vi "KeyInCounterPosition.vi"() -> (1 "Counter Position output":dbl=950.0 min=0.0 max=2600.0 format="%.3f", 2 "Stepper Position":i32)   [LabVIEW 2020]
uses:
  Calibration/GlobalCalLampInfo.vi
  Globals and TypeDefs/gSpectrometer.vi
panel:
  in  "Reset":bool
  in  "Current Wavelength":dbl=703.2413 caption="Input Calibration Wavelength (nm)" format="%.4f"
  in  "Select WL":u16(ring)=5 caption="Select a Target Calibration Line" items=["808.2458  nm  ( Ne )", "794.3181  nm  ( Ne )", "743.8898  nm  ( Ne )", "724.5167  nm  ( Ne )", "717.3938  nm  ( Ne )", "703.2413  nm  ( Ne )", "692.9467  nm  ( Ne )", "671.7043  nm  ( Ne )", "667.8276  nm  ( Ne )", "659.8953  nm  ( Ne )", "653.2882  nm  ( Ne )", "650.6528  nm  ( Ne )", "640.2246  nm  ( Ne )", "638.2991  nm  ( Ne )", "633.4428  nm  ( Ne )", "632.8165  nm  ( Ne )", "579.2200  nm  ( Hg )", "577.1100  nm  ( Hg )", "546.2200  nm  ( Hg )", "435.9500  nm  ( Hg )", "407.8900  nm  ( Hg )", "404.7700  nm  ( Hg )", "366.4300  nm  ( Hg )", "365.5900  nm  ( Hg )", "365.1200  nm  ( Hg )", "Input Wavelength"]
  in  "Cal WL":dbl=514.5 caption="Input Calibration Wavelength (nm)" format="%.4f"
  in  "?":bool
  in  "Counter Position":dbl=7000.0 min=0.0 max=26000.0 format="%.3f"
  # "(nm)"
  # "Find the current wavelength shown on the graph"
  # "(nm)"
  # "Please input your own counter position,\nand then click \"OK\" button."
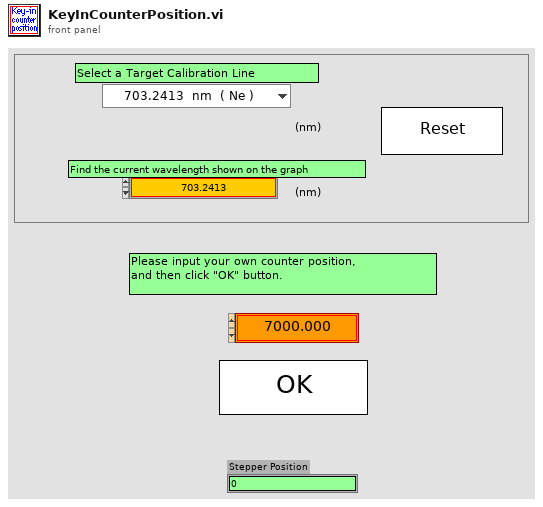
[diagram p1: front panel]
types:
  T1 = cluster{"Element":string, "Wavelength":dbl, "CalWidth":dbl}[]
  T2 = cluster{"Element":string, "Wavelength":dbl, "CalWidth":dbl}
  T3 = typedef "McPherson Grating Density.ctl" = enum8{"150", "300", "600", "1200", "1800"}
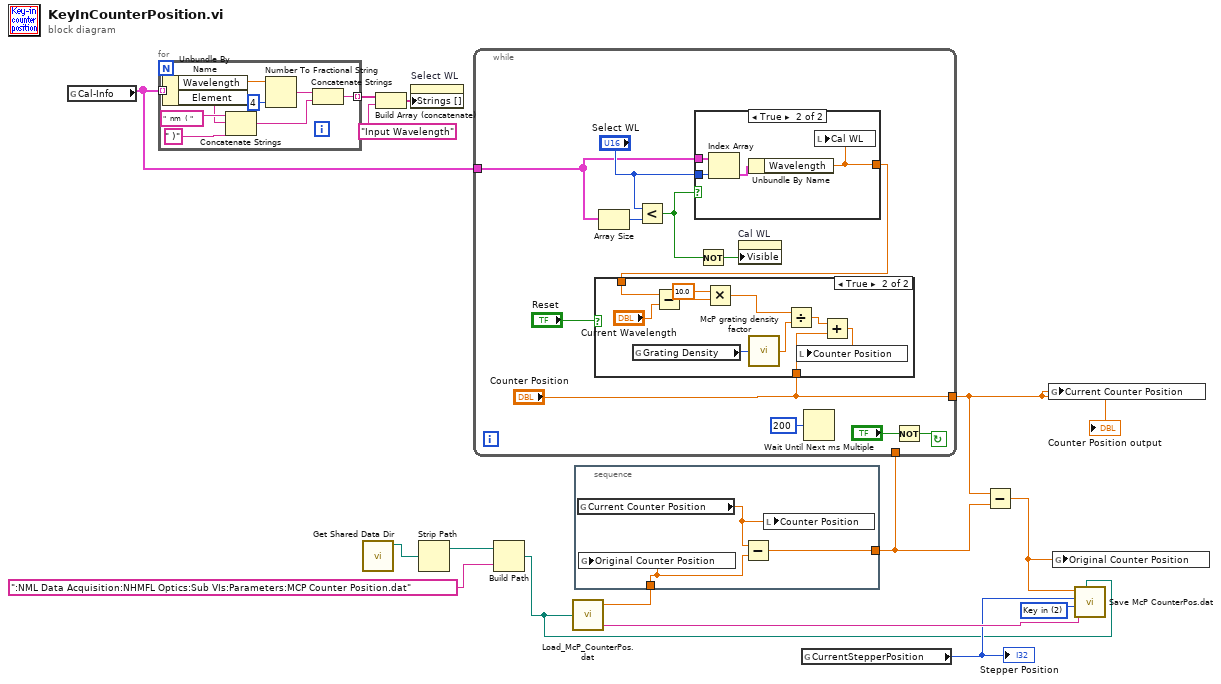
[diagram p0: block diagram]
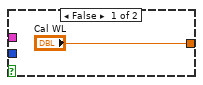
[diagram p3: hidden frame]
diagram:
  w14 = u16 2 items=["Moving", "Calibration", "Key in", "Initialization"] ("Set Method")
  n1 = global read "GlobalCalLampInfo.vi" "Cal-Info"() -> (w5:T1)
  n2 = for {
    tunnel: w5 -> [w24] mode=indexing
    tunnel: [w22] -> w8 mode=indexing
    n3 = Unbundle By Name(w24) -> ("Wavelength"=w21:dbl, "Element"=w18:string)
    n4 = Concatenate Strings("  nm  ( ", w18, " )") -> (w16:string)
    n5 = Number To Fractional String(number=w21, precision (6)=4) -> (F-format string=w20:string)  [unwired: 2 in]
    n6 = Concatenate Strings(w20, w16) -> (w22:string)
  }
  n7 = call "Get Shared Data Dir.vi"() -> ("Data Directory Path"=w3:path)  [unwired: 2 in, 1 out]
  n8 = Build Array (concatenate)(w8, "Input Wavelength") -> (w6:string[])
  n9 = property on="Select WL" class="Ring (strict)"("Strings []"=w6) -> ()  [unwired: 2 in, 2 out]
  n10 = Strip Path(path=w3) -> (stripped path=w4:path)  [unwired: 1 out]
  n11 = Build Path(base path=w4, name or relative path=":NML Data Acquisition:NHMFL Optics:Sub VIs:Parameters:MCP Counter Position.dat") -> (appended path=w2:path)
  n12 = call "Load_McP_CounterPos.dat.VI"("McP Counter Position Path"=w2) -> ("Counter Position"=w12:dbl, "Last Calibration Date"=w15:string)  [unwired: 1 out]
  n13 = stacked-sequence {
    tunnel: [w27] -> w13
    tunnel: w12 -> [w25]
    frame #0 {
      n14 = global read "gSpectrometer.vi" "Current Counter Position"() -> (w26:dbl)
      n15 = global write "gSpectrometer.vi" "Original Counter Position"(w25) -> ()
      n16 = Subtract(x=w26, y=w25) -> (x-y=w27:dbl)
      n17 = local write "Counter Position"(w26) -> ()
    }
  }
  n18 = while {
    tunnel: w13 -> [_]
    tunnel: ["Counter Position"] -> w11
    tunnel: w5 -> [w31]
    stop <- w38 continue-if-true
    n19 = Array Size(array=w31) -> (size(s)=w32:i32)
    n20 = Less?(x="Select WL", y=w32) -> (x < y?=w35:bool)
    n21 = case shown="True" w35 {
      tunnel: ["Cal WL" w51] -> w29
      tunnel: w31 -> [_ w52]
      tunnel: "Select WL" -> [_ w50]
      frame False {
      }
      frame True {
        n22 = Index Array(array=w52, index=w50) -> (element=w53:T2)
        n23 = Unbundle By Name(w53) -> ("Wavelength"=w51:dbl)
        n24 = local write "Cal WL"(w51) -> ()
      }
    }
    n25 = case shown="True" "Reset" {
      tunnel: w29 -> [_ w46]
      tunnel: "Counter Position" -> [_ w40]
      frame False {
      }
      frame True {
        n26 = global read "gSpectrometer.vi" "Grating Density"() -> (w48:T3)
        n27 = Subtract(x=w46, y="Current Wavelength") -> (x-y=w45:dbl)
        n28 = Multiply(x=10.0, y=w45) -> (x*y=w43:dbl)
        n29 = call "McP grating density factor.vi"("Grating Density"=w48) -> ("GratingFactor"=w42:dbl)
        n30 = Divide(x=w43, y=w42) -> (x/y=w41:dbl)
        n31 = Add(x=w41, y=w40) -> (x+y=w39:dbl)
        n32 = local write "Counter Position"(w39) -> ()
      }
    }
    n33 = Not(x=w35) -> (.not. x?=w34:bool)
    n34 = property on="Cal WL" class="DigNum (strict)"("Visible"=w34) -> ()  [unwired: 2 in, 2 out]
    n35 = Wait Until Next ms Multiple(millisecond multiple=u32 200) -> ()  [unwired: 1 out]
    n36 = Not(x="?") -> (.not. x?=w38:bool)
  }
  "Counter Position output" <- w11
  n37 = global read "gSpectrometer.vi" "CurrentStepperPosition"() -> (w9:i32)
  "Stepper Position" <- w9
  n38 = Subtract(x=w11, y=w13) -> (x-y=w10:dbl)
  n39 = global write "gSpectrometer.vi" "Current Counter Position"(w11) -> ()
  n40 = global write "gSpectrometer.vi" "Original Counter Position"(w10) -> ()
  n41 = call "Save McP CounterPos.dat.VI"("McP Counter Position Path"=w2, "Last Calibration Date"=w15, "Set Method"=w14, "McP Stepper Position"=w9, "McP Counter Position"=w10) -> ()  [unwired: 1 in, 1 out]
